vi "GetPositionUm.vi"(8 "error in (no error)":errorcluster, 10 "Stage Label":string, 11 "Stage_MadCityLab in":refnum<class "Stage_MadCityLab.lvclass">) -> (0 "error out":errorcluster, 2 "Stage Position":dbl, 3 "Stage_MadCityLab out":refnum<class "Stage_MadCityLab.lvclass">)   [LabVIEW 2020, in "Stage_MadCityLab.lvlib" / "Stage_MadCityLab.lvclass"]
uses:
  Stage_MadCityLab.lvclass
  Stage_MadCityLab.lvclass/Stage_MadCityLab.ctl
  HAL Layer/Stage/Stage/Stage.lvclass
  Dependency/Madlib.dll
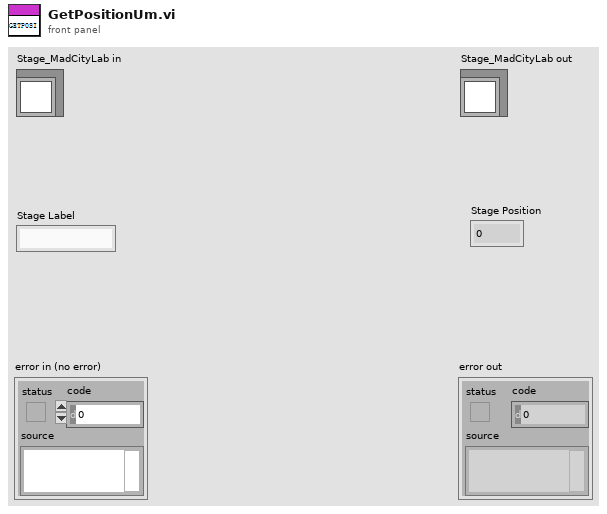
[diagram p1: front panel]
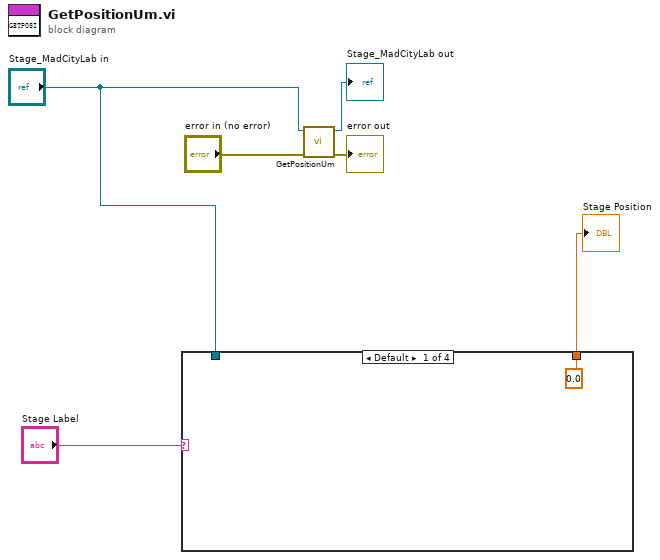
[diagram p0: block diagram]
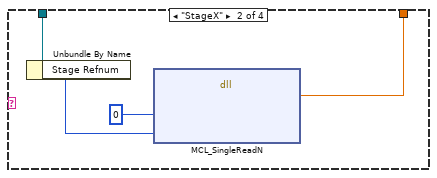
[diagram p2: hidden frame]
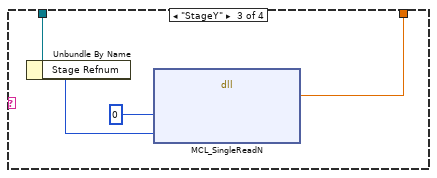
[diagram p3: hidden frame]
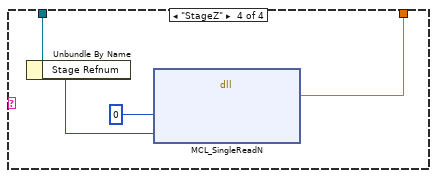
[diagram p4: hidden frame]
diagram:
  n1 = case shown="Default" "Stage Label" {
    tunnel: "Stage_MadCityLab in" -> [_ w11 w15 w19]
    tunnel: [0.0 ("return type") w10 w14 w18] -> w1
    frame Default {
    }
    frame "StageX" {
      n2 = Unbundle By Name(w11) -> ("Stage Refnum"=w9:i32)
      n3 = dll-call lib="E:/Development/DevHardSoftware/MMicroscopyAF/Model/Real Hardware/Stage_MadCityLab/Stage_MadCityLab/Dependency/Madlib.dll" fn="MCL_SingleReadN"("axis"=u32 0, "handle"=w9) -> ("return type"=w10:dbl)  [unwired: 5 in, 2 out]
    }
    frame "StageY" {
      n4 = Unbundle By Name(w15) -> ("Stage Refnum"=w13:i32)
      n5 = dll-call lib="E:/Development/DevHardSoftware/MMicroscopyAF/Model/Real Hardware/Stage_MadCityLab/Stage_MadCityLab/Dependency/Madlib.dll" fn="MCL_SingleReadN"("axis"=u32 0, "handle"=w13) -> ("return type"=w14:dbl)  [unwired: 5 in, 2 out]
    }
    frame "StageZ" {
      n6 = Unbundle By Name(w19) -> ("Stage Refnum"=w17:i32)
      n7 = dll-call lib="E:/Development/DevHardSoftware/MMicroscopyAF/Model/Real Hardware/Stage_MadCityLab/Stage_MadCityLab/Dependency/Madlib.dll" fn="MCL_SingleReadN"("axis"=u32 0, "handle"=w17) -> ("return type"=w18:dbl)  [unwired: 5 in, 2 out]
    }
  }
  "Stage Position" <- w1
  n8 = call-parent "GetPositionUm.vi"("error in (no error)"="error in (no error)", "Stage in"="Stage_MadCityLab in") -> ("error out"=→"error out":errorcluster, "Stage out"=→"Stage_MadCityLab out":refnum<class "Stage_MadCityLab.lvclass">)  [unwired: 7 in, 1 out]
